vi "Heater_Safety.vi"(6 "Ch Names":string[](array[string]), 7 "Values":dbl[](array[numeric]) format="%.2f") -> ()   [LabVIEW 2016]
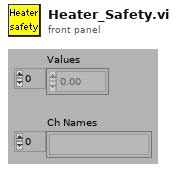
[diagram p1: front panel]
types:
  T1 = typedef "Ch_description_ADAM.ctl" = cluster{"Ch Name":string, "Type":T2, "Function":T3, "Ch State":T4, "Calibration type":T5, "A":dbl, "B":dbl, "C":dbl, "D":dbl, "Comments":string, "Address":T6, "String":string, "Duty":u16}
  T2 = typedef "Module_type_ADAM.ctl" = string
  T3 = typedef "Function_ADAM.ctl" = enum16{"Analogue Input", "Digital Input", "Event counter", "Event rate", "Analogue Output", "Digital Output", "Relay Output"}
  T4 = typedef "Channel_State.ctl" = enum16{"On", "Off", "Always On", "Always Off"}
  T5 = typedef "Calib_type_ADAM.ctl" = string
  T6 = typedef "Address.ctl" = cluster{"Main":i32, "Ch.":i32, "Sub":i32, "Port Name":string}
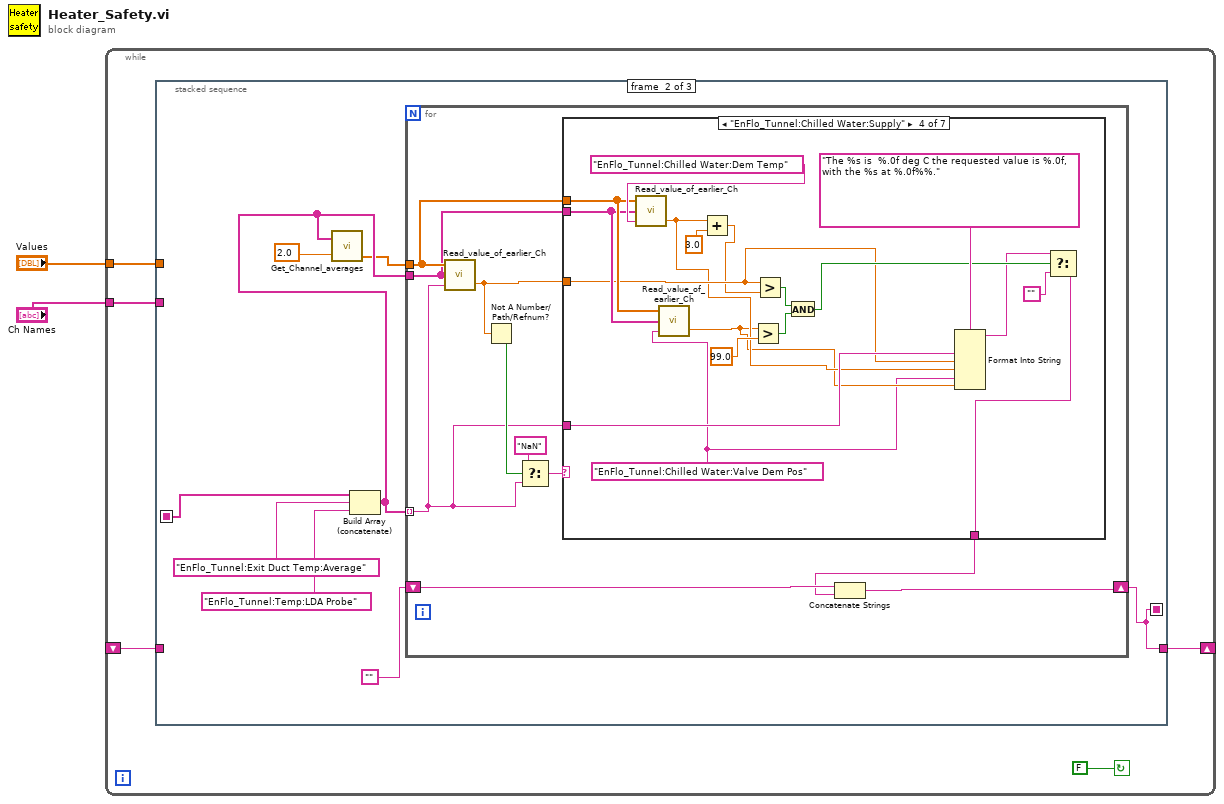
[diagram p0: block diagram]
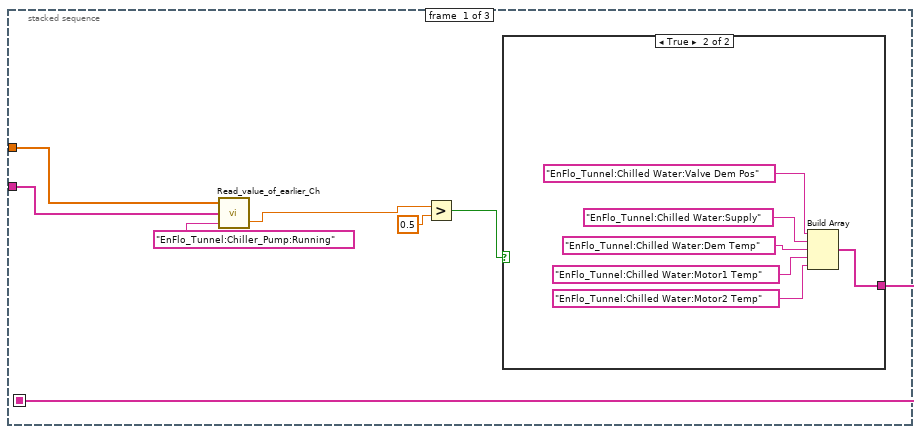
[diagram p2: hidden frame]
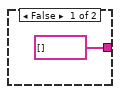
[diagram p3: hidden frame]
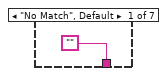
[diagram p4: hidden frame]
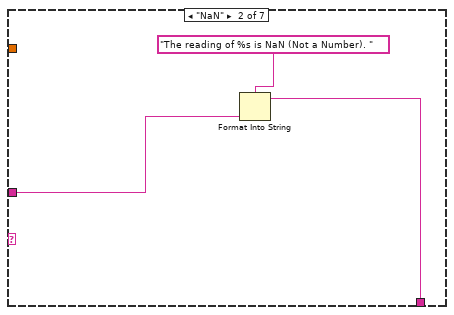
[diagram p5: hidden frame]
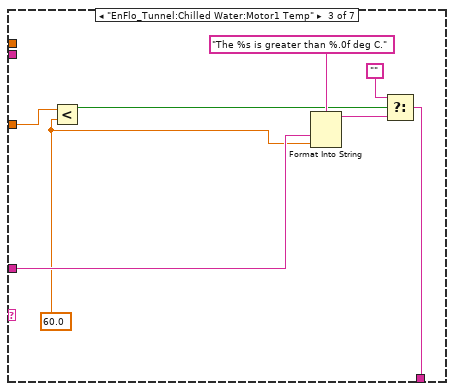
[diagram p6: hidden frame]
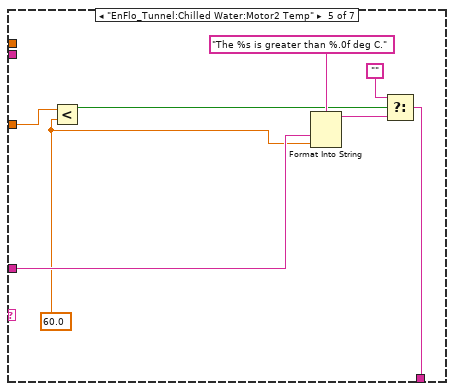
[diagram p7: hidden frame]
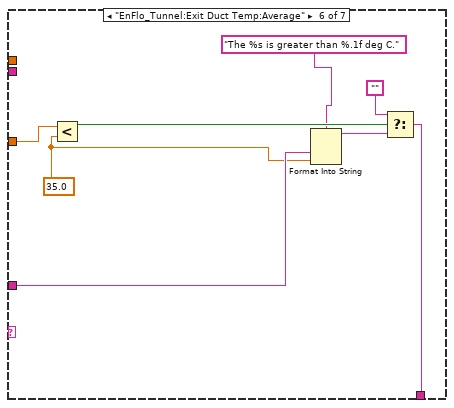
[diagram p8: hidden frame]
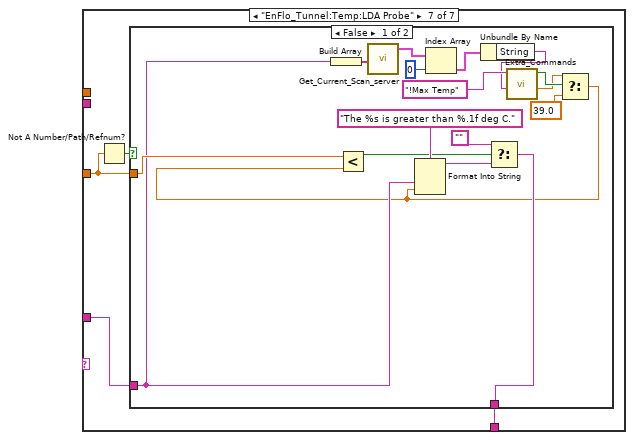
[diagram p9: hidden frame]
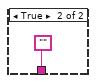
[diagram p10: hidden frame]
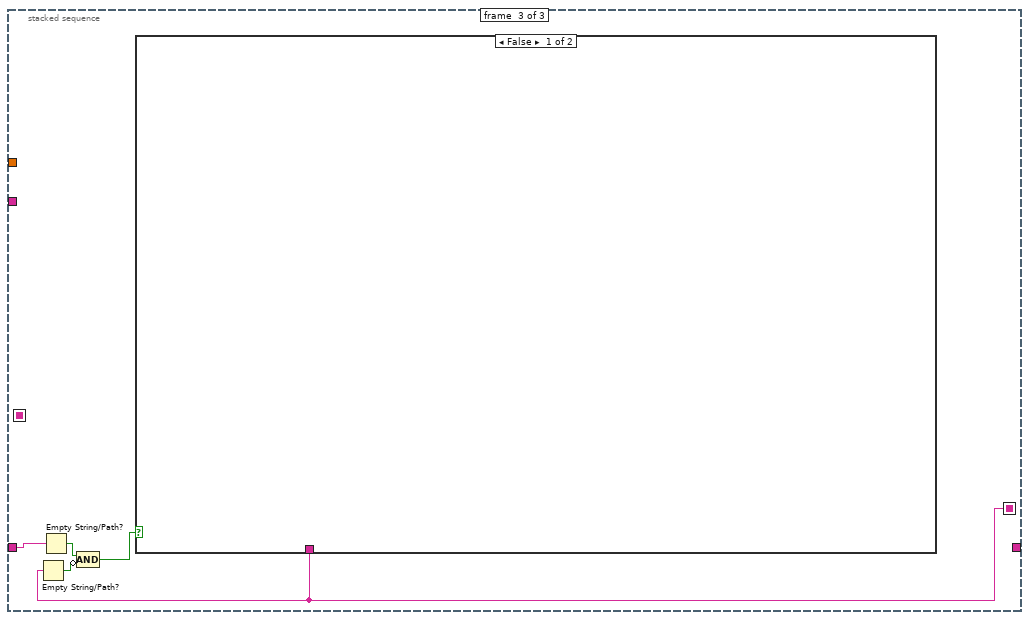
[diagram p11: hidden frame]
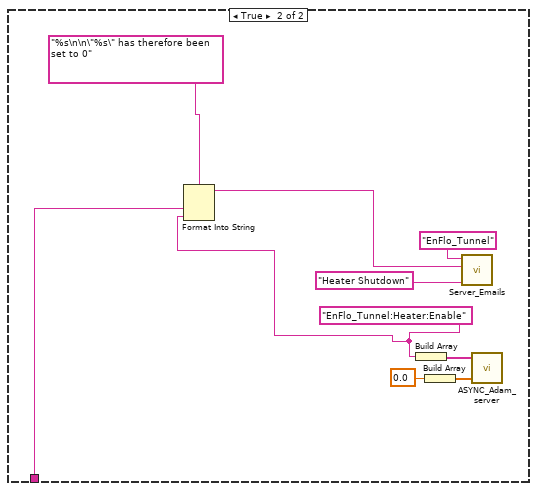
[diagram p12: hidden frame]
diagram:
  n1 = while {
    shift-left: _ -> [w5]
    shift-right: [w6] -> _
    tunnel: "Values" -> [w4]
    tunnel: "Ch Names" -> [w3]
    stop <- FALSE continue-if-true
    n2 = stacked-sequence {
      seq-local: [_ w24 _] -> [_ _ w108]
      seq-local: [w9 _ _] -> [_ w22 _]
      tunnel: [_ w24 _] -> w6
      tunnel: w5 -> [_ _ w112]
      tunnel: w4 -> [w11 _ _]
      tunnel: w3 -> [w10 _ _]
      frame #0 {
        n3 = call "Read_value_of_earlier_Ch.vi"("Desired Ch to Read"="EnFlo_Tunnel:Chiller_Pump:Running", "Ch names"=w10, "Present scan array"=w11) -> ("Value"=w12:dbl)  [unwired: 1 in, 1 out]
        n4 = Greater?(x=w12, y=0.5) -> (0:w8:bool)
        n5 = case shown="True" w8 {
          tunnel: [string[] [] w19] -> w9
          frame False {
          }
          frame True {
            n6 = Build Array("EnFlo_Tunnel:Chilled Water:Valve Dem Pos", "EnFlo_Tunnel:Chilled Water:Supply", "EnFlo_Tunnel:Chilled Water:Dem Temp", "EnFlo_Tunnel:Chilled Water:Motor1 Temp", "EnFlo_Tunnel:Chilled Water:Motor2 Temp") -> (w19:string[])
          }
        }
      }
      frame #1 {
        n7 = Build Array (concatenate)(w22, "EnFlo_Tunnel:Exit Duct Temp:Average", "EnFlo_Tunnel:Temp:LDA Probe") -> (w28:string[])
        n8 = call "Get_Channel_averages.vi"("Desired Ch Names"=w28, "Averaging time (mins)"=2.0) -> ("number"=w25:dbl[])  [unwired: 1 in, 2 out]
        n9 = for {
          tunnel: w28 -> [w30]
          tunnel: w25 -> [w31]
          tunnel: w28 -> [w33] mode=indexing
          shift-right: [w38] -> w24
          shift-left: "" -> [w39]
          n10 = call "Read_value_of_earlier_Ch.vi"("Desired Ch to Read"=w33, "Ch names"=w30, "Present scan array"=w31) -> ("Value"=w36:dbl)  [unwired: 1 in, 1 out]
          n11 = Not A Number/Path/Refnum?(number/path/refnum=w36) -> (NaN/Path/Refnum?=w35:bool)
          n12 = Select(t="NaN", s=w35, f=w33) -> (s? t:f=w32:string)
          n13 = case shown="\"EnFlo_Tunnel:Chilled Water:Supply\"" w32 {
            tunnel: w36 -> [_ _ w51 w56 w77 w81 w87]
            tunnel: w33 -> [_ w41 w50 w69 w76 w85 w89]
            tunnel: ["" w42 w44 w67 w70 w82 w88] -> w37
            tunnel: w31 -> [_ _ _ w64 _ _ _]
            tunnel: w30 -> [_ _ _ w63 _ _ _]
            frame "No Match", Default {
            }
            frame "NaN" {
              n14 = Format Into String(format string="The reading of %s is NaN (Not a Number). " ("Format String"), w41) -> (resulting string=w42:string)  [unwired: 2 in, 1 out]
            }
            frame "EnFlo_Tunnel:Chilled Water:Motor1 Temp" {
              w49 = 60.0 ("y")
              n15 = Less?(x=w51, y=w49) -> (x < y?=w47:bool)
              n16 = Format Into String(format string="The %s is greater than %.0f deg C." ("Format String"), w50, w49) -> (resulting string=w46:string)  [unwired: 2 in, 1 out]
              n17 = Select(t="", s=w47, f=w46) -> (s? t:f=w44:string)
            }
            frame "EnFlo_Tunnel:Chilled Water:Supply" {
              w52 = "EnFlo_Tunnel:Chilled Water:Valve Dem Pos"
              n18 = call "Read_value_of_earlier_Ch.vi"("Desired Ch to Read"="EnFlo_Tunnel:Chilled Water:Dem Temp", "Ch names"=w63, "Present scan array"=w64) -> ("Value"=w54:dbl)  [unwired: 1 in, 1 out]
              n19 = call "Read_value_of_earlier_Ch.vi"("Desired Ch to Read"=w52, "Ch names"=w63, "Present scan array"=w64) -> ("Value"=w53:dbl)  [unwired: 1 in, 1 out]
              n20 = Add(x=w54, y=3.0) -> (x+y=w55:dbl)
              n21 = Greater?(x=w53, y=99.0) -> (0:w61:bool)
              n22 = Greater?(x=w56, y=w55) -> (0:w60:bool)
              n23 = And(x=w60, y=w61) -> (x .and. y?=w59:bool)
              n24 = Format Into String(format string="The %s is  %.0f deg C the requested value is %.0f, with the %s at %.0f%%." ("Format String"), w69, w56, w54, w52, w53) -> (resulting string=w58:string)  [unwired: 2 in, 1 out]
              n25 = Select(t=w58, s=w59, f="") -> (s? t:f=w67:string)
            }
            frame "EnFlo_Tunnel:Chilled Water:Motor2 Temp" {
              w75 = 60.0 ("y")
              n26 = Less?(x=w77, y=w75) -> (x < y?=w73:bool)
              n27 = Format Into String(format string="The %s is greater than %.0f deg C." ("Format String"), w76, w75) -> (resulting string=w72:string)  [unwired: 2 in, 1 out]
              n28 = Select(t="", s=w73, f=w72) -> (s? t:f=w70:string)
            }
            frame "EnFlo_Tunnel:Exit Duct Temp:Average" {
              w84 = 35.0 ("y")
              n29 = Less?(x=w81, y=w84) -> (x < y?=w83:bool)
              n30 = Format Into String(format string="The %s is greater than %.1f deg C." ("Format String"), w85, w84) -> (resulting string=w79:string)  [unwired: 2 in, 1 out]
              n31 = Select(t="", s=w83, f=w79) -> (s? t:f=w82:string)
            }
            frame "EnFlo_Tunnel:Temp:LDA Probe" {
              n32 = Not A Number/Path/Refnum?(number/path/refnum=w87) -> (NaN/Path/Refnum?=w86:bool)
              n33 = case shown="False" w86 {
                tunnel: w87 -> [w106 _]
                tunnel: w89 -> [w100 _]
                tunnel: [w101 ""] -> w88
                frame False {
                  n34 = Build Array(w100) -> (w99:string[])
                  n35 = call "Get_Current_Scan_server.vi"("Desired Channels"=w99) -> ("Ch Description Array"=w98:T1[])  [unwired: 2 out]
                  n36 = Index Array(array=w98, index=0 ("Index")) -> (element=w96:T1)
                  n37 = Unbundle By Name(w96) -> ("String"=w90:string)
                  n38 = call "Extra_Commands.vi"("String to Search"=w90, "Command"="!Max Temp") -> ("Numeric Value"=w93:dbl, "Command Found"=w94:bool)  [unwired: 1 in, 3 out]
                  n39 = Select(t=w93, s=w94, f=39.0) -> (s? t:f=w91:dbl)
                  n40 = Less?(x=w106, y=w91) -> (x < y?=w102:bool)
                  n41 = Format Into String(format string="The %s is greater than %.1f deg C." ("Format String"), w100, w91) -> (resulting string=w104:string)  [unwired: 2 in, 1 out]
                  n42 = Select(t="", s=w102, f=w104) -> (s? t:f=w101:string)
                }
                frame True {
                }
              }
            }
          }
          n43 = Concatenate Strings(w39, w37) -> (w38:string)
        }
      }
      frame #2 {
        n44 = Empty String/Path?(string/path=w108) -> (empty?=w110:bool)
        n45 = Empty String/Path?(string/path=w112) -> (empty?=w111:bool)
        n46 = Compound Arithmetic op=AND(w111, invert w110) -> (w109:bool)
        n47 = case shown="False" w109 {
          tunnel: w108 -> [_ w114]
          frame False {
          }
          frame True {
            w115 = "EnFlo_Tunnel:Heater:Enable"
            n48 = Format Into String(format string="%s\n\n\"%s\" has therefore been set to 0", w114, w115) -> (resulting string=w113:string)  [unwired: 2 in, 1 out]
            n49 = Build Array(w115) -> (w116:string[])
            n50 = Build Array(0.0) -> (w117:dbl[])
            n51 = call "Server_Emails.vi"("Client Name Contains"="EnFlo_Tunnel", "Message"=w113, "Subject"="Heater Shutdown" ("t")) -> ()  [unwired: 2 in, 3 out]
            n52 = call "ASYNC_Adam_server.vi"("Values"=w117, "Channel Names"=w116) -> ()  [unwired: 1 in, 3 out]
          }
        }
      }
    }
  }
